vi "Choreo_TrajectorySwerve_GetInitialSample.vi"(9 "mirrorForRedAlliance":bool, 11 "ChoreoTrajectorySwerve":T2) -> (1 "Exists":bool, 3 "sample":T1={"timestamp"=-999.0, "x"=0.0, "y"=0.0, "heading"=0.0, "velocityX"=0.0, "velocityY"=0.0, "angularVelocity"=0.0, "accelX"=0.0, "accelY"=0.0, "accelAngular"=0.0, "forceX"=[], "forceY"=[]})   [LabVIEW 2019, in "ChoreoLib.lvlib"]
doc: "Create an empty trajectory\n\nInputs: \n <none>\n\nOutputs:\n - ChoreoTrajectory - array - Empty array of Trajectory states."
uses:
  ChoreoLib.lvlib
  TypeDef/ChoreoTrajectorySwerve.ctl
  TypeDef/ChoreoSwerveSample.ctl
  TypeDef/ChoreoEventMarker.ctl
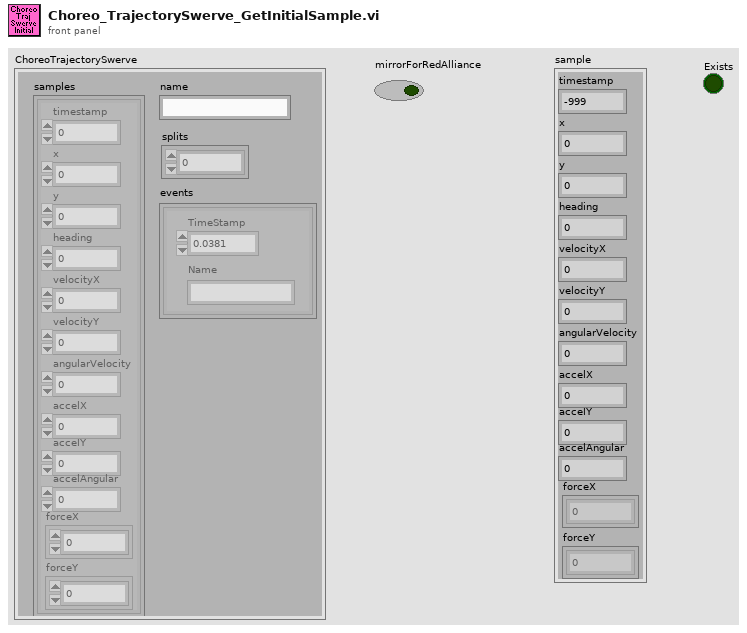
[diagram p1: front panel]
types:
  T1 = typedef "ChoreoLib.lvlib/ChoreoSwerveSample.ctl" = cluster{"timestamp":dbl, "x":dbl, "y":dbl, "heading":dbl, "velocityX":dbl, "velocityY":dbl, "angularVelocity":dbl, "accelX":dbl, "accelY":dbl, "accelAngular":dbl, "forceX":dbl[], "forceY":dbl[]}
  T2 = typedef "ChoreoLib.lvlib/ChoreoTrajectorySwerve.ctl" = cluster{"name":string, "samples":T1[], "splits":i32[], "events":T3[]}
  T3 = typedef "ChoreoLib.lvlib/ChoreoEventMarker.ctl" = cluster{"TimeStamp":dbl, "Name":string}
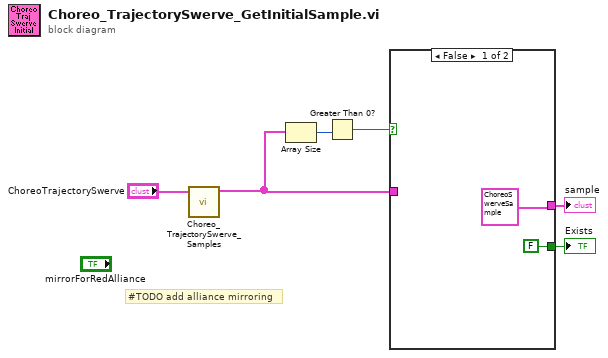
[diagram p0: block diagram]
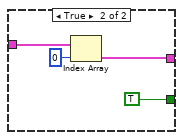
[diagram p2: hidden frame]
diagram:
  # "#TODO add alliance mirroring"
  n1 = call "Choreo_TrajectorySwerve_Samples.vi"("ChoreoTrajectorySwerve"="ChoreoTrajectorySwerve") -> ("samples"=w3:T1[])  [unwired: 10 in]
  n2 = Array Size(array=w3) -> (size(s)=w6:i32)
  n3 = Greater Than 0?(x=w6) -> (x > 0?=w5:bool)
  n4 = case shown="False" w5 {
    tunnel: w3 -> [_ w12]
    tunnel: [T1 {"timestamp"=-999.0, "x"=0.0, "y"=0.0, "heading"=0.0, "velocityX"=0.0, "velocityY"=0.0, "angularVelocity"=0.0, "accelX"=0.0, "accelY"=0.0, "accelAngular"=0.0, "forceX"=[], "forceY"=[]} ("samples") w10] -> w1
    tunnel: [FALSE TRUE] -> w2
    frame False {
    }
    frame True {
      n5 = Index Array(array=w12, index=0) -> (element=w10:T1)
    }
  }
  "Exists" <- w2
  "sample" <- w1
